vi "Delacor_lib_QMH_Dequeue MessageRR.vi"(8 "error in":errorcluster, 9 "timeout in ms (-1)":i32=-1, 11 "Message Queue in":refnum<class "RQMHMessageQueue.lvclass">) -> (0 "error out":errorcluster, 1 "Message Data":variant, 2 "Message":string, 3 "Message Queue out":refnum<class "RQMHMessageQueue.lvclass">, 5 "Reply":T1)   [LabVIEW 2024, in "RQMHMessageQueue.lvclass"]
doc: "This VI pulls messages off the Message Queue.\n____\nDQMH Framework: Palette 7.1.0.1503\nCopyright (c) 2025, DQMH Consortium"
uses:
  RQMHMessageQueue.lvclass
  JQMHCore/Module/Reply.ctl
  RQMHMessageQueue.lvclass/RQMHMessageQueue.ctl
  JQMHCore/Module/RQMHModule.lvclass
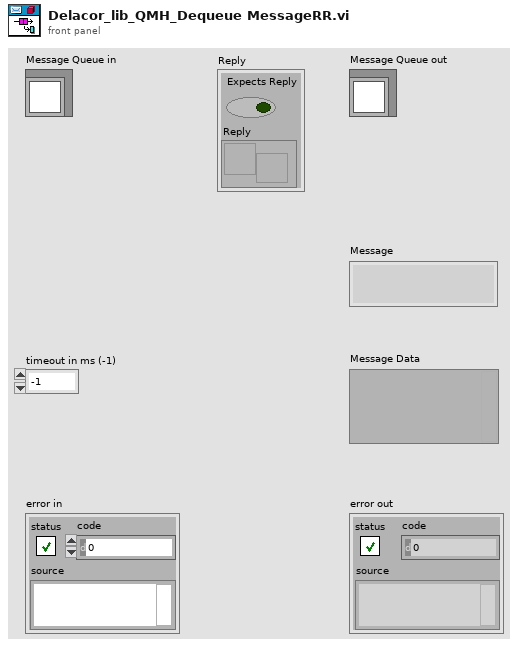
[diagram p1: front panel]
types:
  T1 = typedef "RQMHModule.lvclass/Reply.ctl" = cluster{"Expects Reply":bool, "Reply":refnum<notifier>}
  T2 = cluster{"Message Data":variant, "Reply Payload":T1}
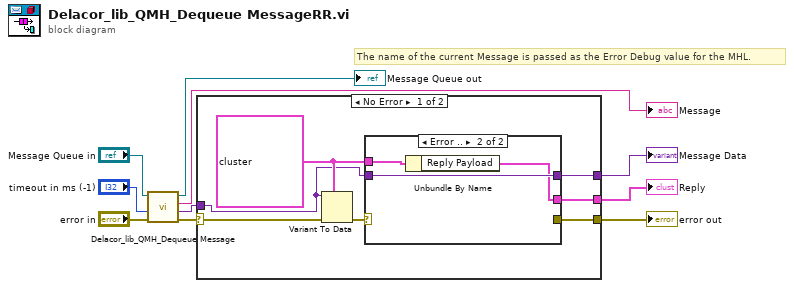
[diagram p0: block diagram]
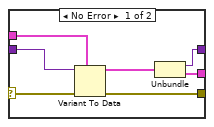
[diagram p2: hidden frame]
diagram:
  # "The name of the current Message is passed as the Error Debug value for the MHL."
  n1 = call-dynamic "Delacor_lib_QMH_Dequeue Message.vi"("error in"="error in", "timeout in ms (-1)"="timeout in ms (-1)", "Message Queue in"="Message Queue in") -> ("error out"=w1:errorcluster, "Message Data"=w5:variant, "Message"=→"Message":string, "Message Queue out"=→"Message Queue out":refnum<class "RQMHMessageQueue.lvclass">)  [unwired: 5 in]
  n2 = case shown="No Error" w1 {
    selector: w1 -> [w11 w28]
    tunnel: w5 -> [w15 _]
    tunnel: [w14 w28] -> w4
    tunnel: [w13 _] -> w3
    tunnel: [w12 _] -> w2
    frame No Error {
      w16 = T2 {"Message Data"=variant, "Reply Payload"={"Expects Reply"=FALSE, "Reply"=refnum}} ("cluster")
      n3 = Variant To Data(error in=w11, type=w16, Variant=w15) -> (error out=w17:errorcluster)  [unwired: 1 out]
      n4 = case shown="Error .." w17 {
        selector: w17 -> [w24 _]
        tunnel: w16 -> [w23 w26]
        tunnel: w15 -> [w22 w27]
        tunnel: [w21 _] -> w14
        tunnel: [w19 w27] -> w13
        tunnel: [w18 w25] -> w12
        frame No Error {
          n5 = Variant To Data(error in=w24, type=w23, Variant=w22) -> (data=w20:T2, error out=w21:errorcluster)
          n6 = Unbundle(w20) -> ("Message Data"=w19:variant, "Reply Payload"=w18:T1)
        }
        frame Error {
          n7 = Unbundle By Name(w26) -> ("Reply Payload"=w25:T1)
        }
      }
    }
    frame Error {
    }
  }
  "error out" <- w4
  "Message Data" <- w3
  "Reply" <- w2
